vi "getUnits.vi"(8 "error in (no error)":errorcluster, 10 "channelName":string, 11 "StaticOutputEditor in":refnum<class "StaticOutputEditor.lvclass">) -> (0 "error out":errorcluster, 2 "units":string, 3 "StaticOutputEditor out":refnum<class "StaticOutputEditor.lvclass">)   [LabVIEW 2011, in "Views.lvlib" / "ScriptEditor.lvlib" / "StaticOutputEditor.lvclass"]
uses:
  StaticOutputEditor.lvclass
  StaticOutputEditor.lvclass/StaticOutputEditor.ctl
  Tools/DatabaseHelpers/Database Objects/ChannelArray/ChannelArray.lvclass
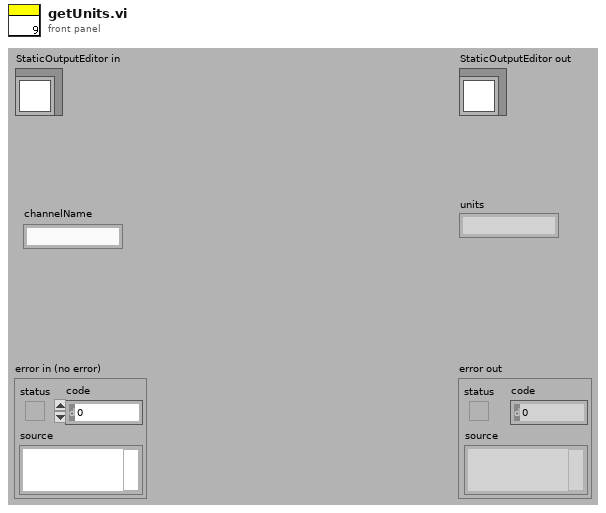
[diagram p1: front panel]
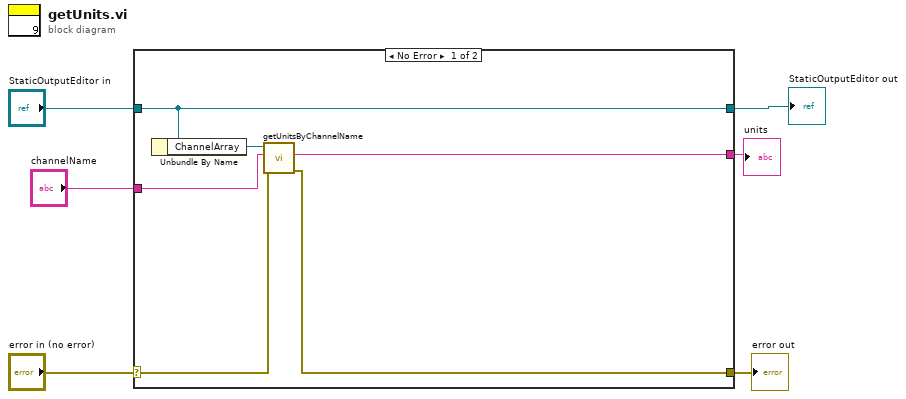
[diagram p0: block diagram]
diagram:
  n1 = case shown="No Error" "error in (no error)" {
    selector: "error in (no error)" -> [w9 w14]
    tunnel: [w8 w14] -> w5
    tunnel: [w12 w13] -> w3
    tunnel: "StaticOutputEditor in" -> [w12 w13]
    tunnel: "channelName" -> [w10 _]
    tunnel: [w7 _] -> w1
    frame No Error {
      n2 = Unbundle By Name(w12) -> ("ChannelArray"=w11:refnum<class "ChannelArray.lvclass">)
      n3 = call "getUnitsByChannelName.vi"("error in (no error)"=w9, "channel_name"=w10, "ChannelArray in"=w11) -> ("error out"=w8:errorcluster, "units"=w7:string)  [unwired: 6 in, 1 out]
    }
    frame Error {
    }
  }
  "error out" <- w5
  "StaticOutputEditor out" <- w3
  "units" <- w1
